vi "TL2100LAB05.vi"() -> ()   [LabVIEW 2020]
panel:
  out "Pump Status":bool
  out "Height, cm":dbl(slide) scale=0.0..60.0
  out "System Status":bool
  out "Low Pressure":bool
  out "kPa":dbl(knob) scale=0.0..7.0 scale format="%.0g"
  out "in(H2O)":dbl(knob) scale=0.0..25.0
  out "AtoD":i16 format="%04x"
  out "Volts":dbl(knob) scale=1.0..5.0
  in  "stop":bool
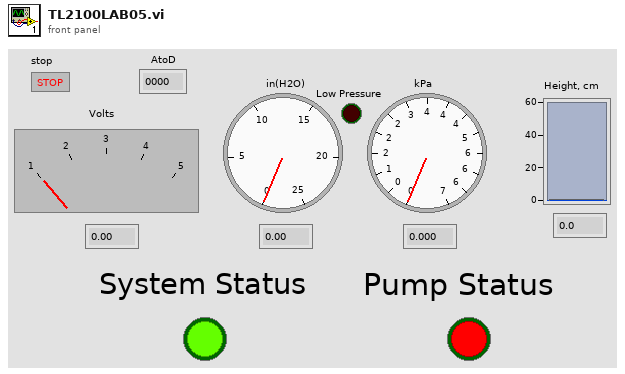
[diagram p1: front panel]
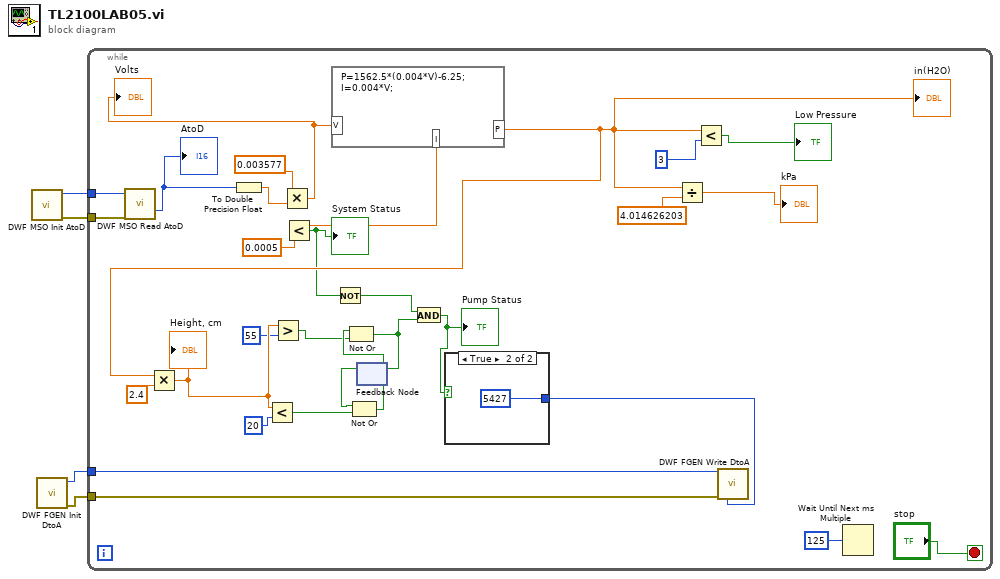
[diagram p0: block diagram]
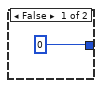
[diagram p2: hidden frame]
diagram:
  n1 = call "DWF MSO Init AtoD.vi"() -> ("Error Out"=w3:errorcluster, "Instrument Handle Out"=w4:u32)  [unwired: 10 in]
  n2 = call "DWF FGEN Init DtoA.vi"() -> ("Error Out"=w1:errorcluster, "Instrument Handle Out"=w2:u32)  [unwired: 10 in]
  n3 = while {
    tunnel: w4 -> [w34]
    tunnel: w3 -> [w33]
    tunnel: w2 -> [w11]
    tunnel: w1 -> [w10]
    stop <- "stop" stop-if-true
    n4 = call "DWF MSO Read AtoD.vi"("Instrument Handle In AtoD"=w34, "Error In"=w33) -> ("AtoD"=w29:i16)  [unwired: 12 in, 1 out]
    "AtoD" <- w29
    n5 = To Double Precision Float(number=w29) -> (double precision float=w28:dbl)
    n6 = Multiply(x=0.003577, y=w28) -> (x*y=w27:dbl)
    "Volts" <- w27
    n7 = formula code="P=1562.5*(0.004*V)-6.25;\nI=0.004*V;"("V"=w27) -> ("P"=w19:dbl, "I"=w21:dbl)
    "in(H2O)" <- w19
    n8 = Multiply(x=w19, y=2.4) -> (x*y=w13:dbl)
    "Height, cm" <- w13
    n9 = Less?(x=w13, y=20) -> (x < y?=w14:bool)
    n10 = Greater?(x=w13, y=55) -> (0:w16:bool)
    n11 = Less?(x=w21, y=0.0005) -> (x < y?=w6:bool)
    "System Status" <- w6
    n12 = Not(x=w6) -> (.not. x?=w7:bool)
    n13 = feedback #1() -> (w17:bool)  [unwired: 1 in]
    n14 = Not Or(1:w14, 2:w17) -> (0:w18:bool)
    n15 = Not Or(1:w16, 2:w18) -> (0:w8:bool)
    n16 = feedback-in #1(w8) -> ()
    n17 = And(x=w7, y=w8) -> (x .and. y?=w5:bool)
    "Pump Status" <- w5
    n18 = case shown="True" w5 {
      tunnel: [0 5427] -> w9
      frame False {
      }
      frame True {
      }
    }
    n19 = Divide(x=w19, y=4.014626203) -> (x/y=→"kPa":dbl)
    n20 = Less?(x=w19, y=3) -> (x < y?=→"Low Pressure":bool)
    n21 = call "DWF FGEN Write DtoA.vi"("Instrument Handle In"=w11, "Error In"=w10, "Raw Data"=w9) -> ()  [unwired: 11 in, 2 out]
    n22 = Wait Until Next ms Multiple(millisecond multiple=125) -> ()  [unwired: 1 out]
  }
